vi "analyse.vi"(1 "Array":dbl[](array[numeric])) -> (0 "Cluster":T1)   [LabVIEW 2025]
uses:
  <vilib>/Analysis/baseanly.llb/Mean (DBL).vi
  <vilib>/Analysis/NI_AALBase.lvlib
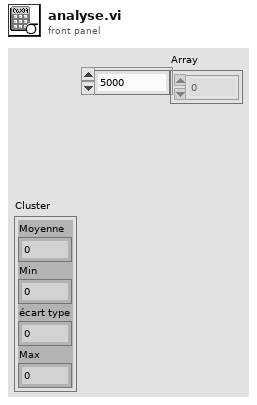
[diagram p1: front panel]
types:
  T1 = cluster{"Moyenne":dbl, "Min":dbl, "écart type":dbl, "Max":dbl}
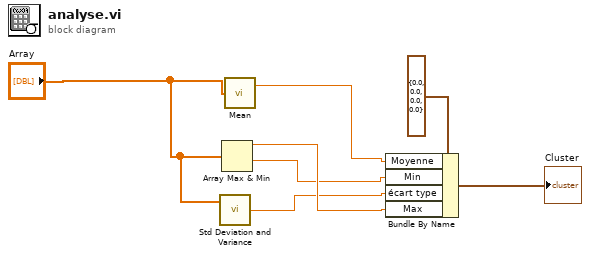
[diagram p0: block diagram]
diagram:
  n1 = call <vilib>:"Std Deviation and Variance.vi"("X"="Array") -> ("standard deviation"=w4:dbl)  [unwired: 1 in, 2 out]
  n2 = Array Max & Min(array="Array") -> (max value=w6:dbl, min value=w5:dbl)  [unwired: 2 out]
  n3 = call-poly <vilib>:"Mean.vi"("X"="Array") -> ("mean"=w7:dbl)  [unwired: 1 out]
  n4 = Bundle By Name(cluster=T1 {"Moyenne"=0.0, "Min"=0.0, "écart type"=0.0, "Max"=0.0} ("input cluster"), "Moyenne"=w7, "Min"=w5, "écart type"=w4, "Max"=w6) -> (→"Cluster":T1)
